vi "Update Time Entry.vi"(8 "error in (no error)":errorcluster, 11 "Time Entries in":refnum<class "Time Entries.lvclass">) -> (0 "error out":errorcluster, 3 "Time Entries out":refnum<class "Time Entries.lvclass">)   [LabVIEW 2020, in "Time Entries.lvclass"]
uses:
  Time Entries.lvclass
  Time Entries.lvclass/Time Entries.ctl
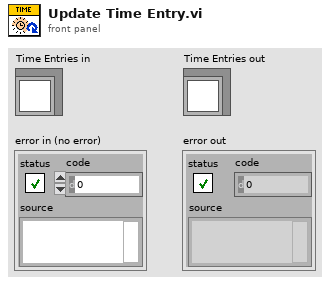
[diagram p1: front panel]
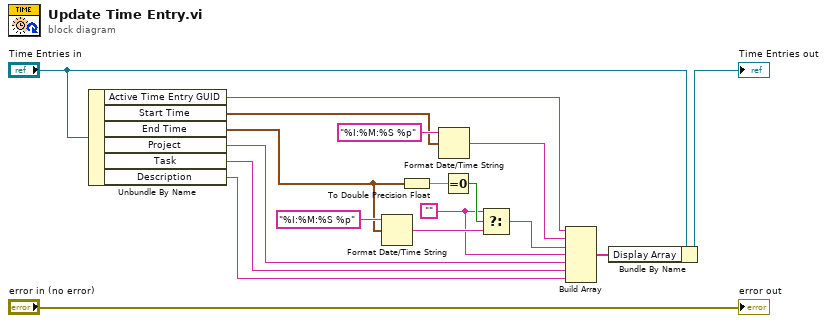
[diagram p0: block diagram]
diagram:
  w1 = ""
  n1 = Unbundle By Name("Time Entries in") -> ("Active Time Entry GUID"=w12:string, "Start Time"=w11:timestamp, "End Time"=w6:timestamp, "Project"=w5:string, "Task"=w4:string, "Description"=w3:string)
  n2 = Format Date/Time String(time format string (%c)="%I:%M:%S %p", seconds (now)=w6) -> (date/time string=w9:string)  [unwired: 1 in]
  n3 = To Double Precision Float(number=w6) -> (double precision float=w8:dbl)
  n4 = Format Date/Time String(time format string (%c)="%I:%M:%S %p", seconds (now)=w11) -> (date/time string=w15:string)  [unwired: 1 in]
  n5 = Equal To 0?(x=w8) -> (x = 0?=w7:bool)
  n6 = Select(t=w1, s=w7, f=w9) -> (s? t:f=w2:string)
  n7 = Build Array(w12, w15, w2, w1, w5, w4, w3) -> (w14:string[])
  n8 = Bundle By Name(cluster="Time Entries in", "Display Array"=w14) -> (→"Time Entries out":refnum<class "Time Entries.lvclass">)
  "error out" <- "error in (no error)"
